vi "Test Next Empty Correct for Empty Suite.vi"(8 "error in (no error)":errorcluster, 11 "Test Case In":refnum<class "Runnable Next Test.lvclass">) -> (0 "error out":errorcluster, 3 "Test Case Out":refnum<class "Runnable Next Test.lvclass">)   [LabVIEW 2020, in "Runnable Next Test.lvclass"]
uses:
  Runnable Next Test.lvclass
  C:/Program Files (x86)/National Instruments/LabVIEW 2020/vi.lib/Astemes/LUnit/Test Case.lvclass
  <vilib>/Astemes/LUnit/Test Case.lvclass/Test Case.ctl
  e8c5eeff-a694-4c0d-b261-74e2e6f5327d.vi
  <vilib>/Astemes/LUnit/Append Pass Result.vi
  <vilib>/Astemes/LUnit/Append Fail Result.vi
  <vilib>/Astemes/LUnit/Compare Variants.vi
  <vilib>/Astemes/LUnit/Describe Comparison.vi
  <vilib>/Astemes/LUnit/Variant to string.vi
  <vilib>/Utility/Data Type/Get Type Information.vi
  <vilib>/Utility/LVClass/Get LV Class Name.vi
  source/API/LUnit Test Suite/LUnit Test Suite.lvclass
  Runnable Next Test.lvclass/Runnable Next Test.ctl
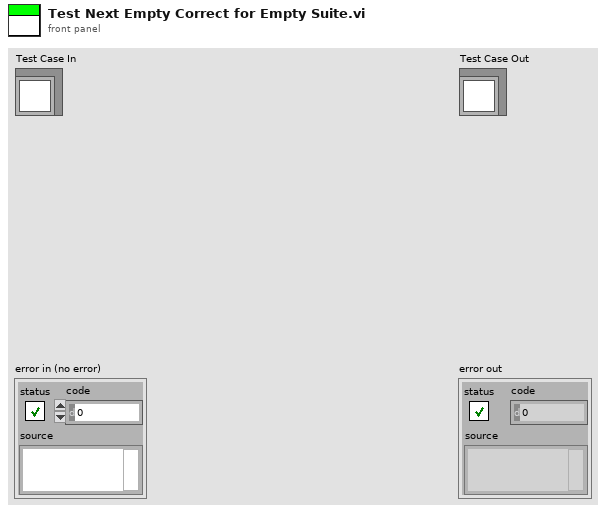
[diagram p1: front panel]
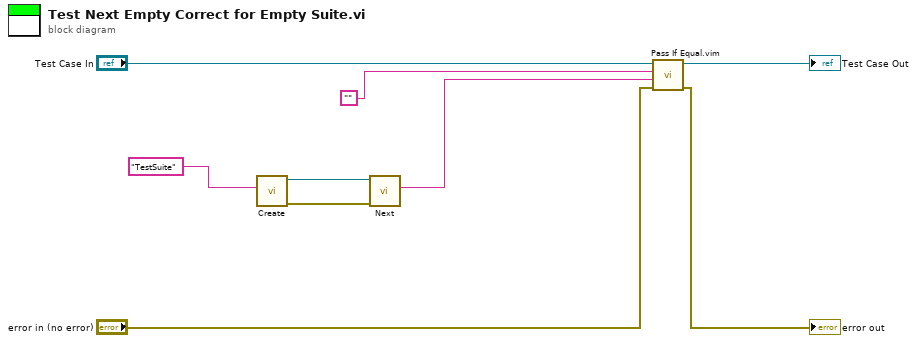
[diagram p0: block diagram]
diagram:
  n1 = call "Create.vi"("Suite Name"="TestSuite") -> ("error out"=w5:errorcluster, "LUnit Test Suite Out"=w4:refnum<class "LUnit Test Suite.lvclass">)  [unwired: 9 in]
  n2 = call-dynamic "Next.vi"("error in (no error)"=w5, "LUnit Test Suite In"=w4) -> ("Name"=w2:string)  [unwired: 6 in, 3 out]
  n3 = call "Pass If Equal.vim"("error in (no error)"="error in (no error)", "Actual"=w2, "Expected"="", "LUnit Test Case In"="Test Case In") -> ("error out"=→"error out":errorcluster, "LUnit Test Case Out"=→"Test Case Out":refnum<class "Runnable Next Test.lvclass">)  [unwired: 6 in]
